vi "例6-2.vi"() -> ()   [LabVIEW 2019]
uses:
  <vilib>/Analysis/NI_AALBase.lvlib
panel:
  in  "停止":bool
  in  "信号类型":enum16{"正弦波", "三角波", "方波", "锯齿波"}(ring)
  in  "采样点数":dbl=1000.0
  in  "采样频率":dbl=1000.0
  in  "方波占空比":dbl=50.0
  in  "初始相位":dbl
  in  "信号幅度":dbl=1.0
  in  "信号频率":dbl=5.0
  out "波形图":cluster{i32, dbl, "sine wave":dbl[]}(graph)
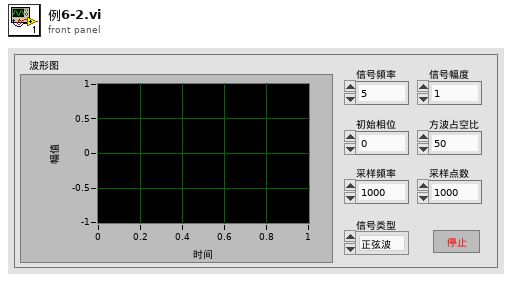
[diagram p1: front panel]
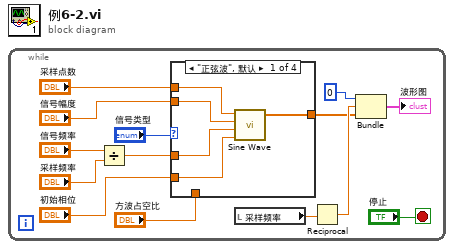
[diagram p0: block diagram]
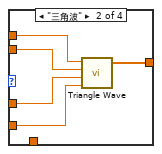
[diagram p2: hidden frame]
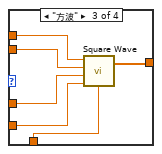
[diagram p3: hidden frame]
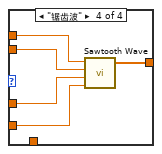
[diagram p4: hidden frame]
diagram:
  n1 = while {
    stop <- "停止" stop-if-true
    n2 = Divide(x="信号频率", y="采样频率") -> (x/y=w9:dbl)
    n3 = case shown="\"正弦波\", 默认" "信号类型" {
      tunnel: "采样点数" -> [w19 w23 w29 w34]
      tunnel: "信号幅度" -> [w18 w22 w28 w33]
      tunnel: w9 -> [w17 w21 w27 w32]
      tunnel: "初始相位" -> [w16 w20 w26 w31]
      tunnel: [w15 w24 w30 w35] -> w4
      tunnel: "方波占空比" -> [_ _ w25 _]
      frame "正弦波", Default {
        n4 = call <vilib>:"Sine Wave.vi"("samples"=w19, "amplitude"=w18, "frequency"=w17, "phase in"=w16) -> ("sine wave"=w15:dbl[])  [unwired: 1 in, 2 out]
      }
      frame "三角波" {
        n5 = call <vilib>:"Triangle Wave.vi"("samples"=w23, "amplitude"=w22, "frequency"=w21, "phase in"=w20) -> ("triangle wave"=w24:dbl[])  [unwired: 1 in, 2 out]
      }
      frame "方波" {
        n6 = call <vilib>:"Square Wave.vi"("samples"=w29, "amplitude"=w28, "frequency"=w27, "duty cycle (%)"=w25, "phase in"=w26) -> ("square wave"=w30:dbl[])  [unwired: 1 in, 2 out]
      }
      frame "锯齿波" {
        n7 = call <vilib>:"Sawtooth Wave.vi"("samples"=w34, "amplitude"=w33, "frequency"=w32, "phase in"=w31) -> ("sawtooth wave"=w35:dbl[])  [unwired: 1 in, 2 out]
      }
    }
    n8 = local read "采样频率"() -> (w6:dbl)
    n9 = Reciprocal(x=w6) -> (1/x=w5:dbl)
    n10 = Bundle(0, w5, "sawtooth wave"=w4) -> (→"波形图":cluster{i32, dbl, "sawtooth wave":dbl[]})  [unwired: 1 in]
  }
